vi "CSM - State Table - DebugTool.vi"() -> ()   [LabVIEW 2017]
doc: "<In Development> Real-time status table for the entire CSM program module."
uses:
  _Support/Typedef/_CSM_GlobalLog_MSG_TYPE.ctl
  _Support/Typedef/_CSM_GlobalLog_MSG.ctl
  _Support/Typedef/_CSM_Response Source Message.ctl
  _Polymophic/Add State(s) to Queue By BOOL(Element).vi
  76e8844a-bf39-49de-bef4-434369a066cd.vi
  e359954a-2527-40a5-9e0b-778f8f2f97ef.vi
  _Support/GlobalEvent/Gevt-ThreadQueueName.vi
  <vilib>/Utility/config.llb/Close Config Data.vi
  <vilib>/Utility/config.llb/Write Key.vi
  <vilib>/Utility/config.llb/Write Key (Double).vi
  <vilib>/Utility/config.llb/Write Key (I32).vi
  <vilib>/Utility/config.llb/Write Key (Path).vi
  <vilib>/Utility/config.llb/Write Key (String).vi
  <vilib>/Utility/config.llb/Write Key (Boolean).vi
  <vilib>/Utility/Data Type/Get Type Information.vi
  <vilib>/Utility/config.llb/Open Config Data.vi
  _csmHelper/lvcsmFile/lvcsm File Path.vi
  <vilib>/Utility/config.llb/Read Key.vi
  <vilib>/Utility/config.llb/Read Key (Double).vi
  <vilib>/Utility/config.llb/Read Key (I32).vi
  <vilib>/Utility/config.llb/Read Key (Path).vi
  <vilib>/Utility/config.llb/Read Key (String).vi
  <vilib>/Utility/config.llb/Read Key (Boolean).vi
  Communicable State Machine.lvlib
  _Support/csm-tool-support.lvlib
panel:
  in  "LogSize Limit:":i32=4 min=4 step=1
  out "ModuleNum:":i32=4 min=4 max=20 step=1
  out "LogSize:":i32=2 min=2 max=10 step=1
  in  "Content":string[][](array[string])
  in  "Row Header Strings[]":string[](array[string])
  in  "Exit":bool
  in  "Clear CSM":bool
  out "Table":string[][](table)
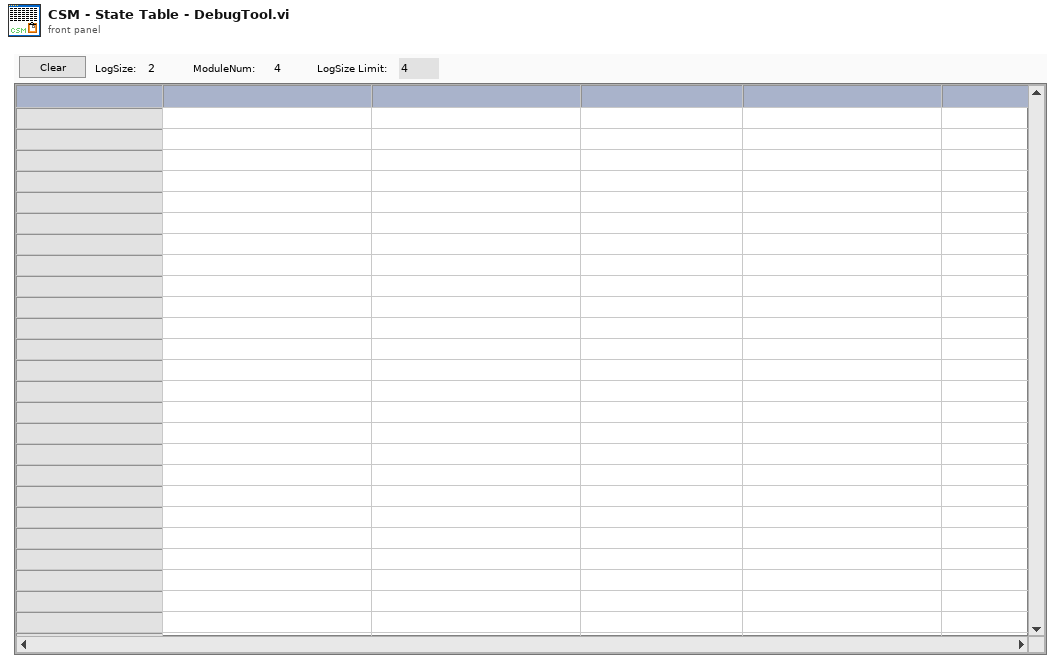
[diagram p1: front panel]
types:
  T1 = typedef "Communicable State Machine.lvlib/_CSM_GlobalLog_MSG_TYPE.ctl" = enum16{"User Log", "State Change", "Status", "Interrupt", "Register", "Unregister", "Error Log", "Module Created", "Module Destroyed"}
  T2 = enum32{"Invalid", "Standard", "Closed", "Hidden", "Minimized", "Maximized"}
  T3 = enum32{"invalid app kind", "Development System", "Run Time System", "Student Edition", "Embedded LabVIEW", "Evaluation", "Custom"}
  T4 = typedef "Communicable State Machine.lvlib/_CSM_GlobalLog_MSG.ctl" = cluster{"Name(\"\" to use uuid)":string, "Current State":string, "Arguments":string, "Source Message":T5, "Source Module":string, "Complete(T)/Start(F)":bool, "LogType":T1}
  T5 = typedef "Communicable State Machine.lvlib/_CSM_Response Source Message.ctl" = cluster{"‘State":string, "’Arguments":string, "’Error":errorcluster}
  T6 = cluster{"Core":cluster{"Current VI Reference":refnum<vi>, "Close Panel on Exit?":bool}, "Global-DataTable":string[][], "LogSize Limit":i32, "CSM Global Log Event":refnum<user-event>, "Log":T4, "LogTime":timestamp, "JKISM Names":string[], "RowHeaders":string[], "Content":string[][]}
  T7 = cluster{"Current VI Reference":refnum<vi>, "Close Panel on Exit?":bool}
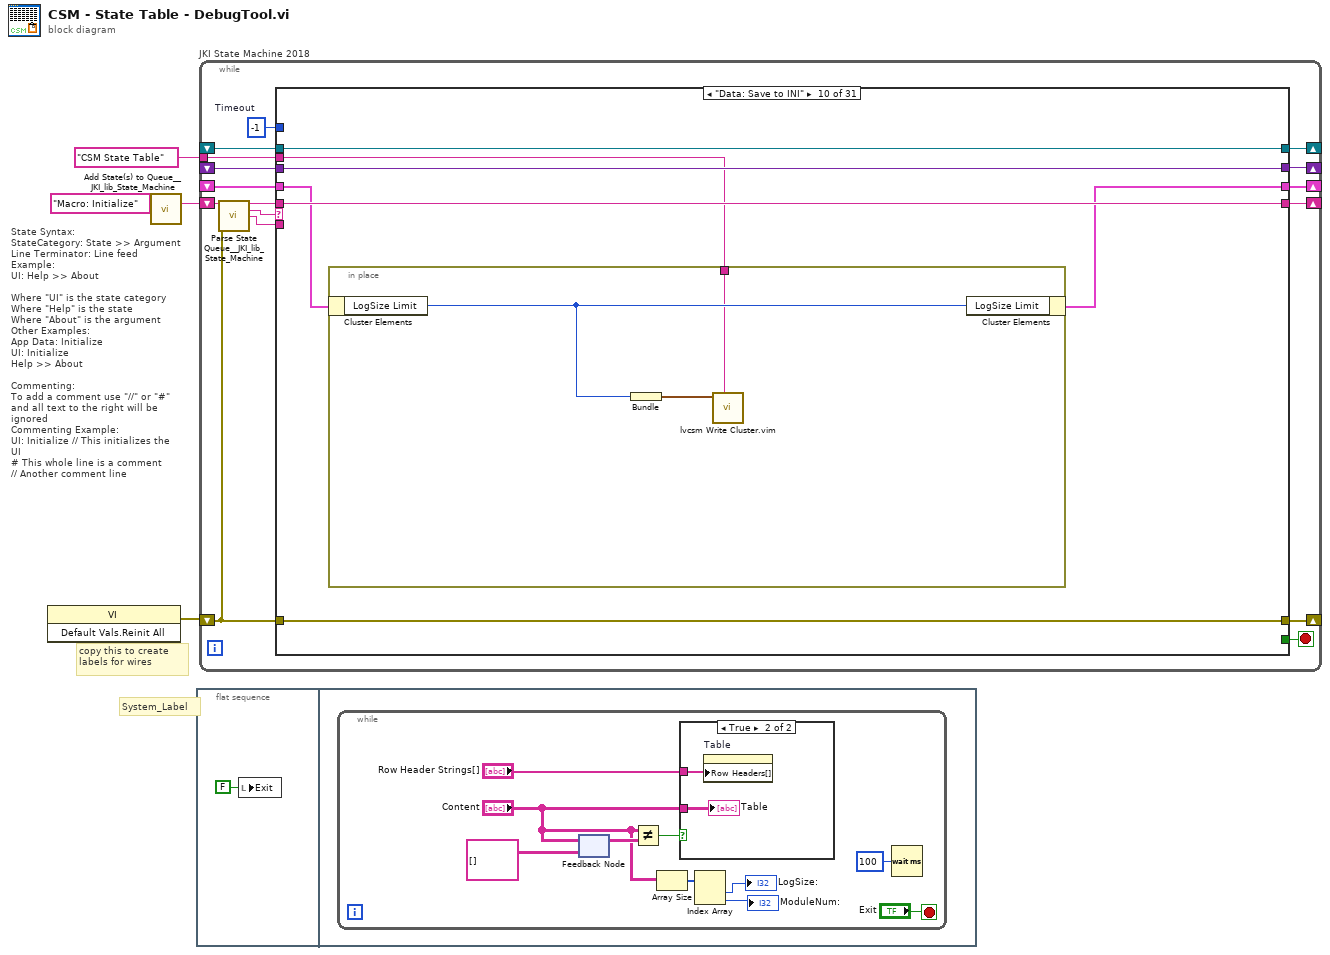
[diagram p0: block diagram]
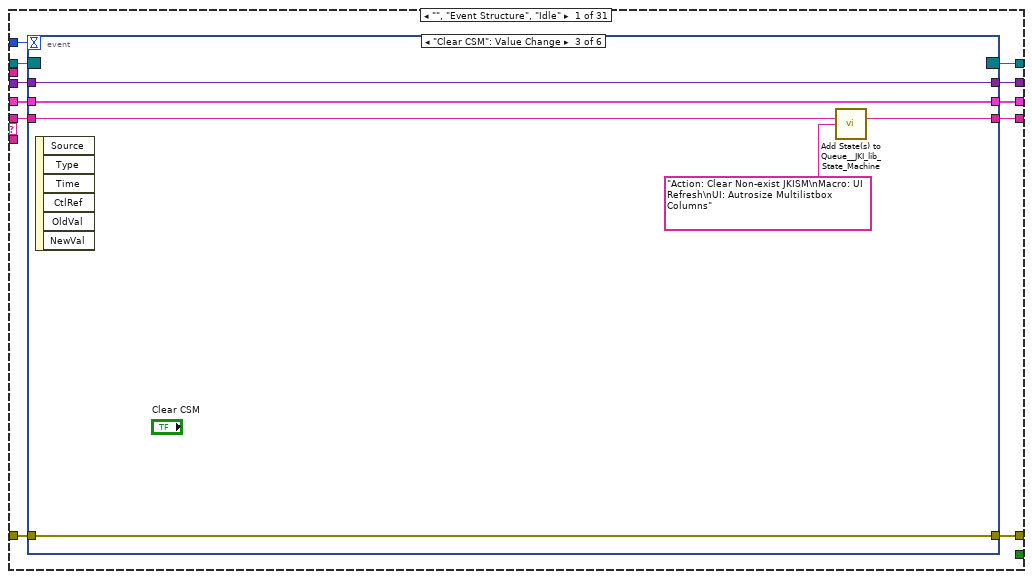
[diagram p3: hidden frame]
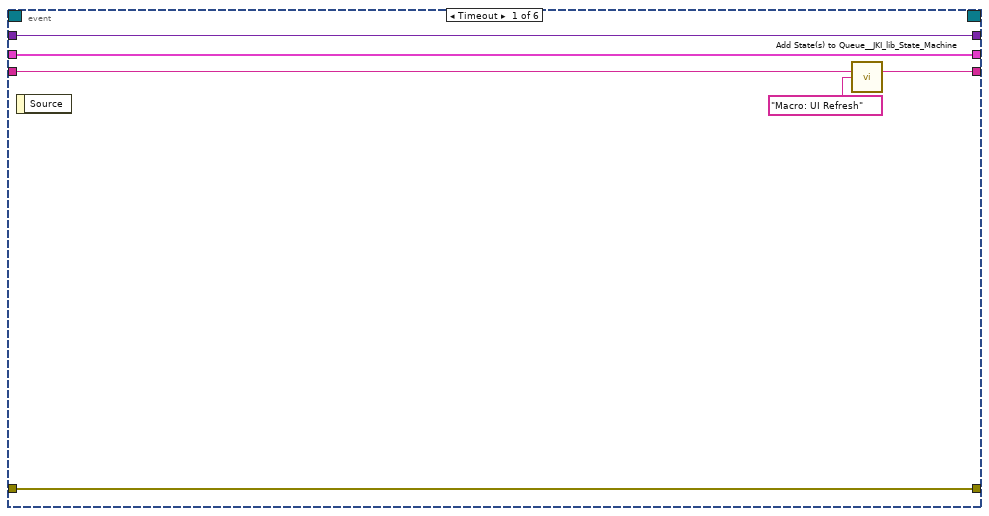
[diagram p4: hidden frame]
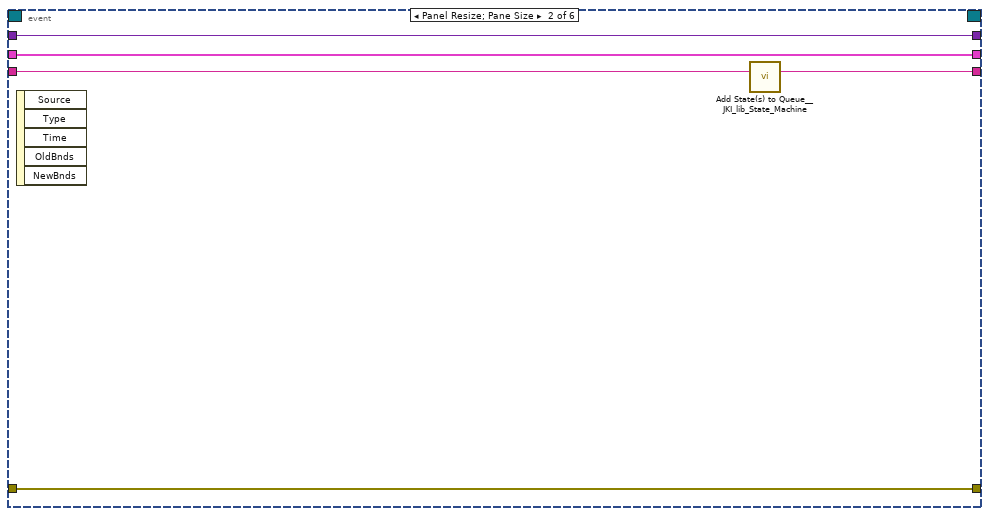
[diagram p5: hidden frame]
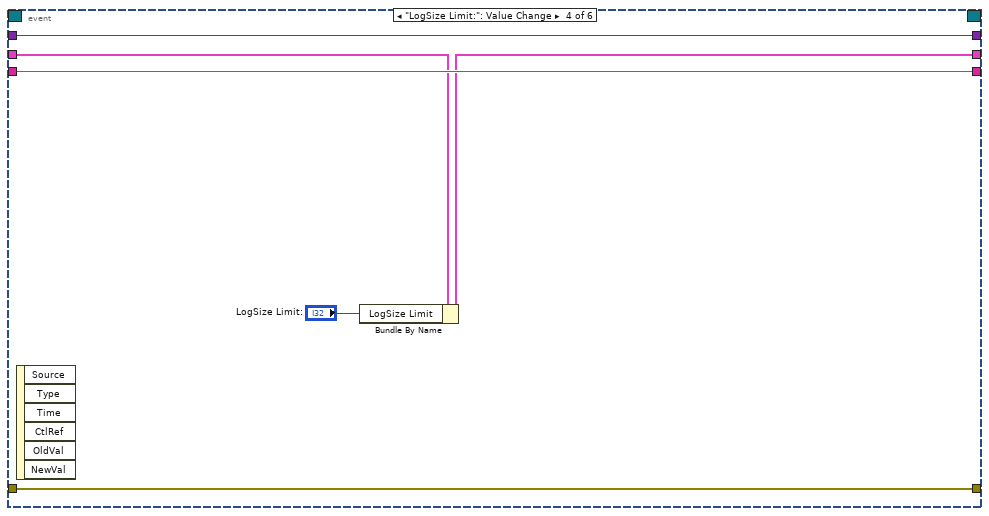
[diagram p6: hidden frame]
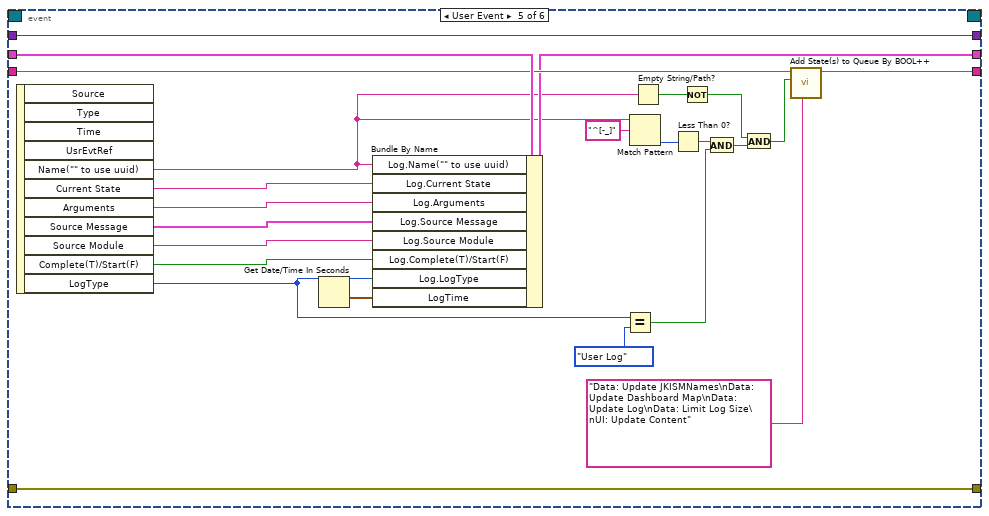
[diagram p7: hidden frame]
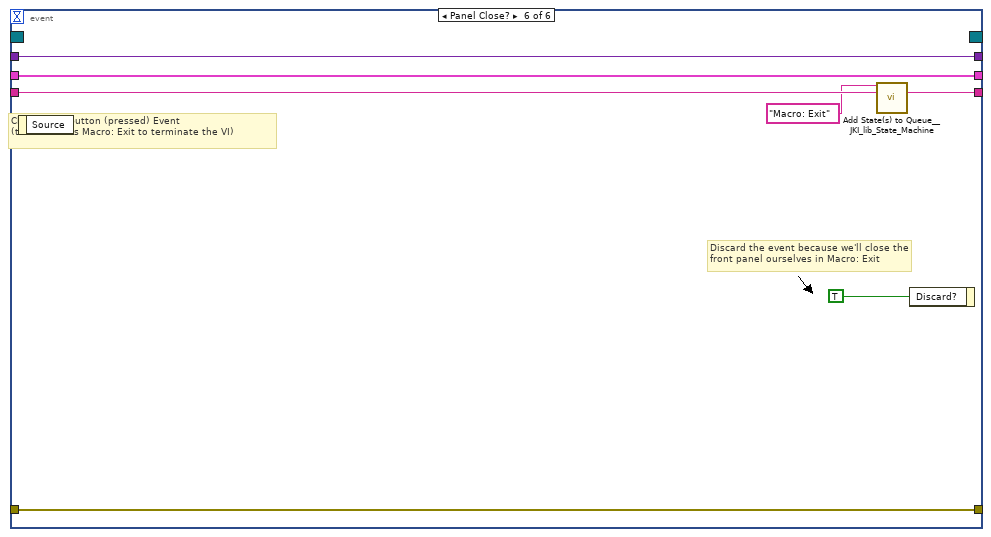
[diagram p8: hidden frame]
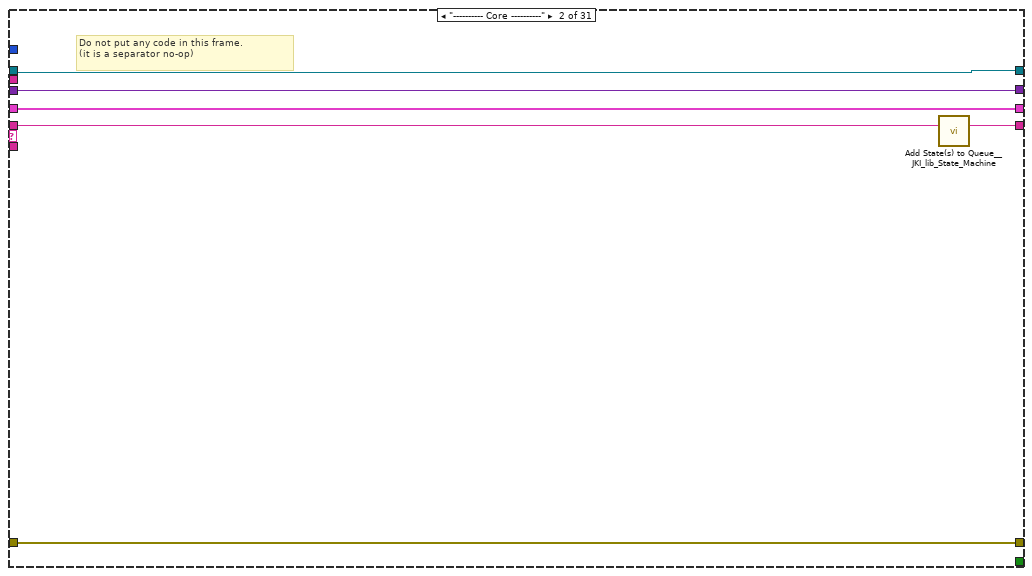
[diagram p9: hidden frame]
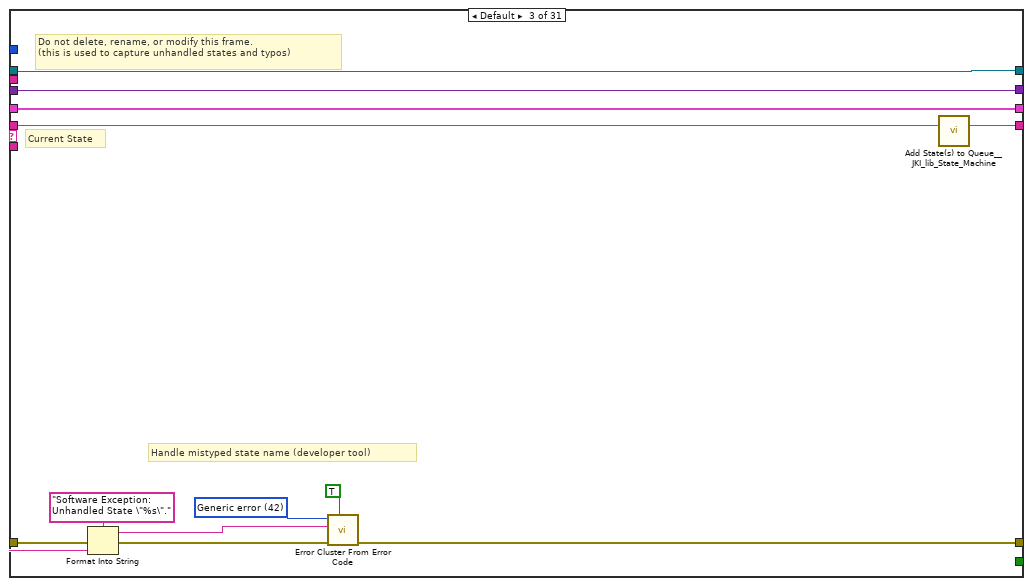
[diagram p10: hidden frame]
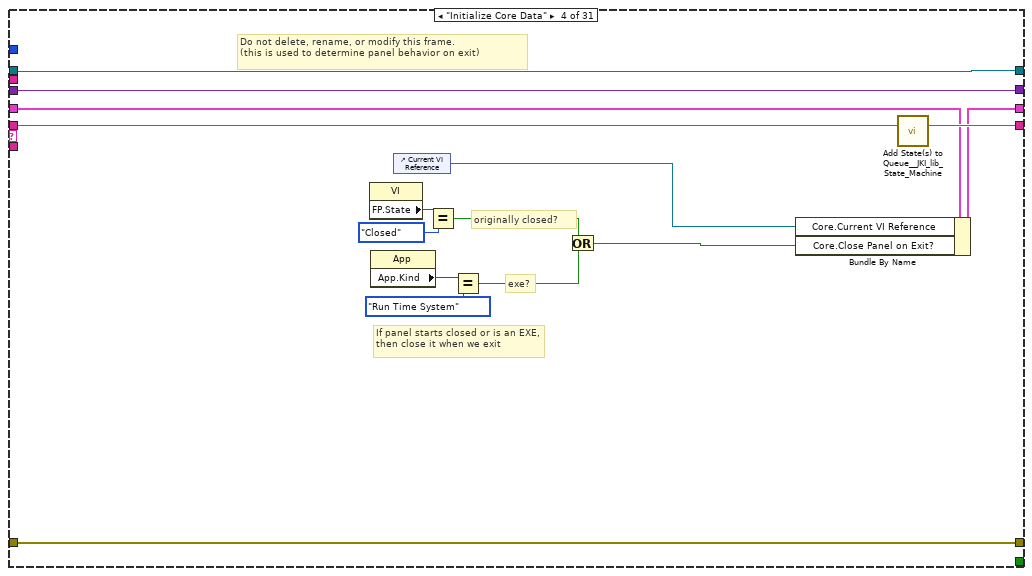
[diagram p11: hidden frame]
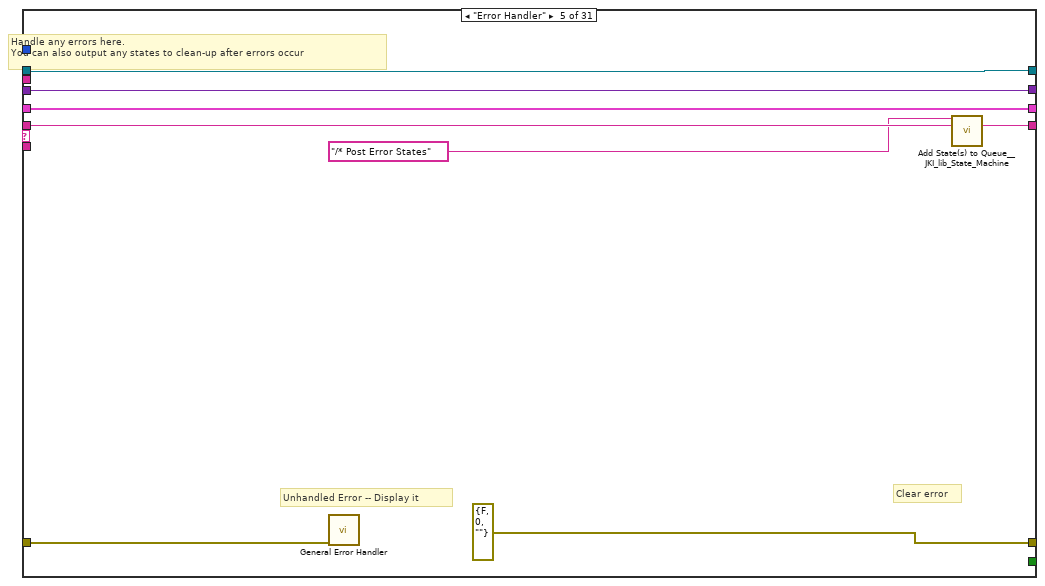
[diagram p12: hidden frame]
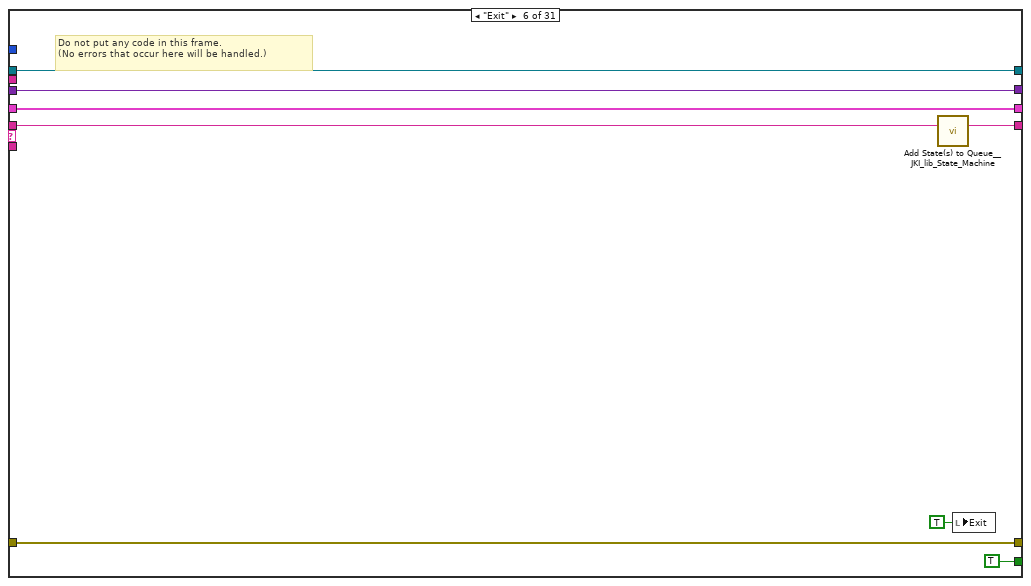
[diagram p13: hidden frame]
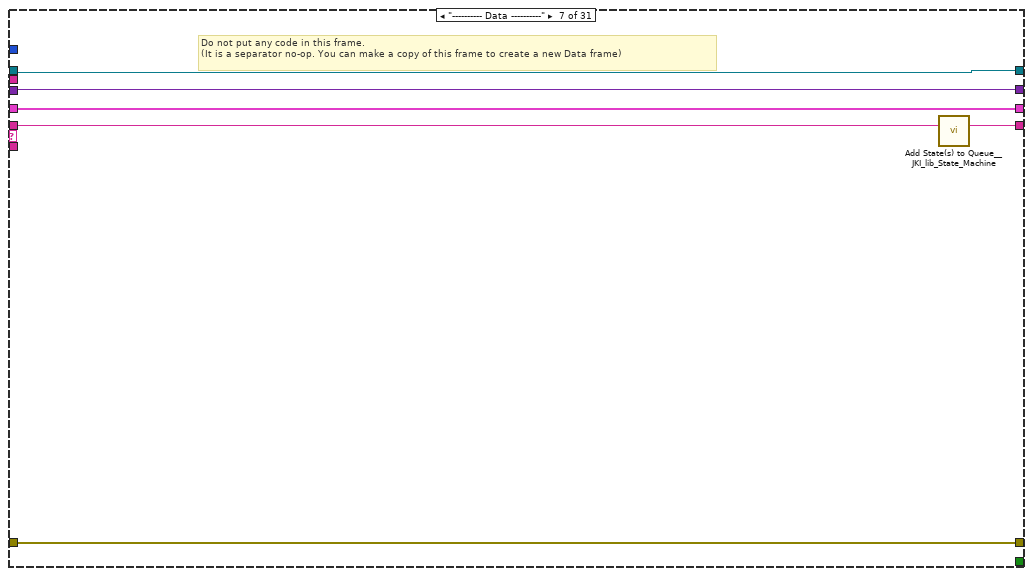
[diagram p14: hidden frame]
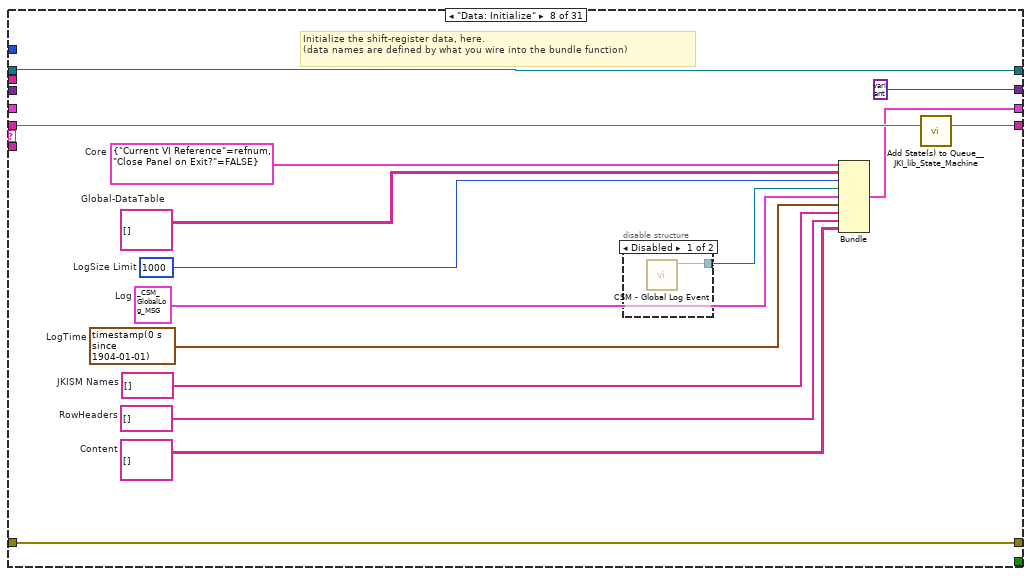
[diagram p15: hidden frame]
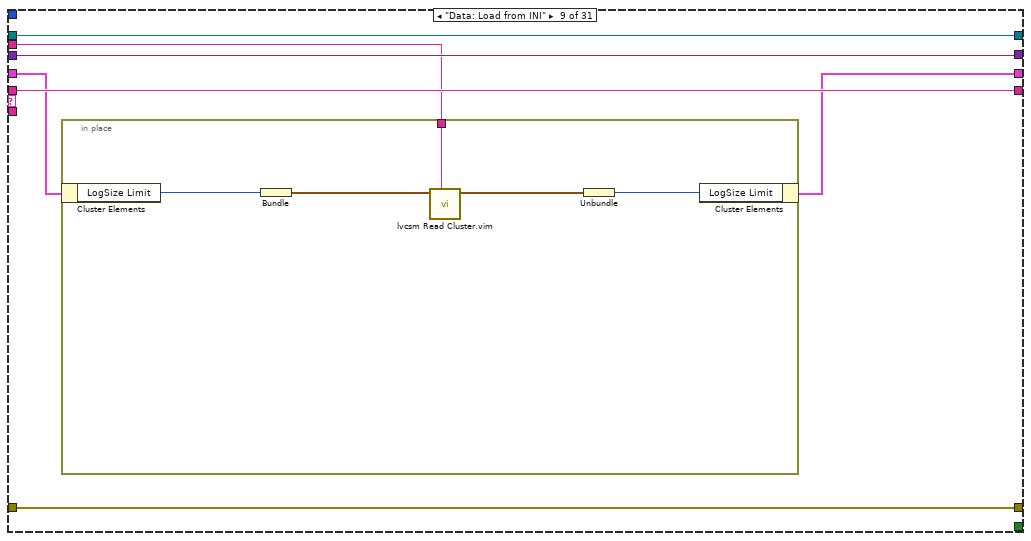
[diagram p17: hidden frame]
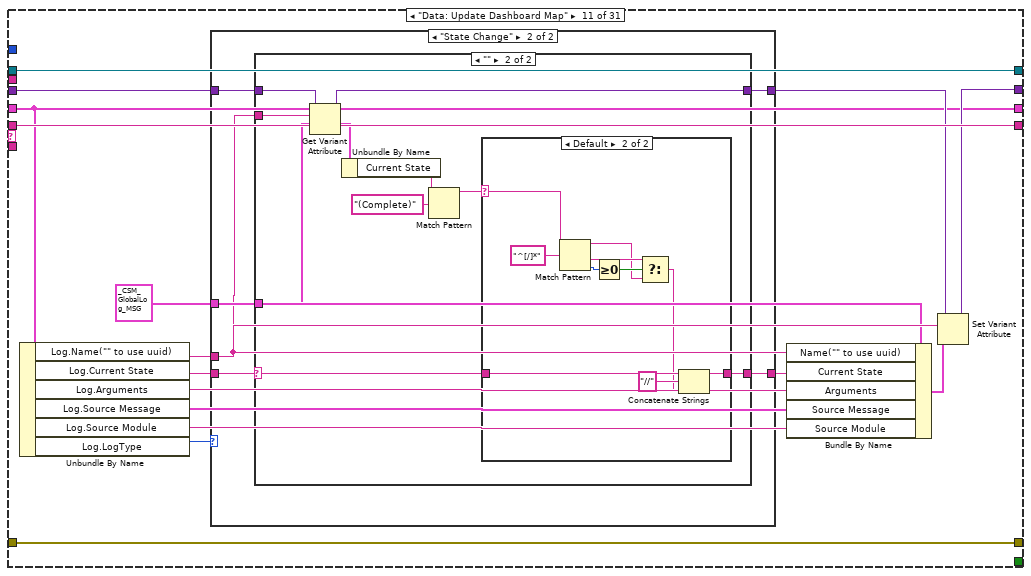
[diagram p18: hidden frame]
diagram:
  # "State Syntax:\nStateCategory: State >> Argument\nLine Terminator: Line feed\nExample:\nUI: Help >> About\n\nWhere \"UI\" is the state category\nWhere \"Help\" is the state\nWhere \"About\" is the argument\nOther Examples:\nApp Data: Initialize\nUI: Initialize\nHelp >> About\n\nCommenting:\nTo add a comment use \"//\" or \"#\" and all text to the right will be ignored\nCommenting Example:\nUI: Initialize // This initializes the UI\n# This whole line is a comment\n// Another comment line"
  # "copy this to create labels for wires"
  # "System_Label"
  n1 = invoke class="VI" method="Default Vals.Reinit All"() -> (error out=w2:errorcluster)  [unwired: 3 in, 2 out]
  n2 = call <vilib>:"Add State(s) to Queue__JKI_lib_State_Machine.vi"("State(s) in (\"\")"="Macro: Initialize") -> ("States Out"=w3:string)  [unwired: 14 in]
  n3 = flat-sequence {
    frame #0 {
      n4 = local write "Exit"(FALSE ("Exit")) -> ()
    }
    frame #1 {
      n5 = while {
        stop <- "Exit" stop-if-true
        n6 = feedback-in #1("Content") -> ()
        n7 = feedback #1(string[][] [] ("Content")) -> (w11:string[][])
        n8 = Not Equal?(x="Content", y=w11) -> (x != y?=w12:bool)
        n9 = Array Size(array="Content") -> (size(s)=w8:i32[])
        n10 = case shown="True" w12 {
          tunnel: "Content" -> [_ w17]
          tunnel: "Row Header Strings[]" -> [_ w16]
          frame False {
          }
          frame True {
            n11 = property on="Table" class="Tbl (strict)"("Row Headers[]"=w16) -> ()  [unwired: 2 in, 2 out]
            "Table" <- w17
          }
        }
        n12 = Index Array(array=w8) -> (element #1=→"LogSize:":i32, element #2=→"ModuleNum:":i32)  [unwired: 2 in]
        n13 = Wait (ms)(milliseconds to wait=u32 100) -> ()  [unwired: 1 out]
      }
    }
  }
  n14 = while "JKI State Machine 2018" {
    shift-right: [w26] -> _
    shift-left: _ -> [w25]
    shift-right: [w29] -> _
    shift-left: w2 -> [w23]
    shift-right: [w28] -> _
    shift-left: w3 -> [w30]
    shift-right: [w22] -> _
    shift-left: _ -> [w21]
    shift-right: [w20] -> _
    shift-left: _ -> [w19]
    tunnel: "CSM State Table" ("key") -> [w18]
    stop <- w27 stop-if-true
    w24 = -1  # Timeout
    n15 = call <vilib>:"Parse State Queue__JKI_lib_State_Machine.vi"("State Queue"=w30, "Error In (no error)"=w23) -> ("Remaining States"=w32:string, "Current State"=w33:string, "Arguments"=w31:string)  [unwired: 11 in]
    n16 = case shown="\"Data: Save to INI\"" w33 {
      selector: w33 -> [_ _ w107 _ _ _ _ _ _ _ _ _ _ _ _ _ _ _ _ _ _ _ _ _ _ _ _ _ _ _ _]
      tunnel: w32 -> [w44 w104 w111 w132 w140 w148 w154 w169 w176 w188 w207 w250 w281 w300 w316 w322 w330 w338 w351 w421 w428 w436 w440 w448 w456 w463 w470 w478 w491 w495 w520]
      tunnel: w31 -> [_ _ _ _ _ _ _ _ _ _ _ _ _ _ _ _ _ w333 w345 _ _ _ _ _ _ _ _ _ _ _ _]
      tunnel: w25 -> [w42 w101 w109 w125 w137 w146 w151 _ w175 w187 w195 w244 w277 w297 w311 w319 w324 w336 w347 w418 w425 w433 w439 w447 w452 w460 w467 w473 w488 w494 w511]
      tunnel: [w41 w102 w113 w129 errorcluster {"status"=FALSE, "code"=0, "source"=""} ("error out") w145 w152 w165 w177 w189 w208 w251 w282 w301 w310 w320 w328 w334 w348 w422 w429 w430 w441 w449 w457 w461 w468 w476 w489 w496 w521] -> w29
      tunnel: w23 -> [w40 w102 w112 w129 w136 w145 w152 w165 w177 w189 w208 w251 w282 w301 w313 w320 w328 w335 w349 w422 w429 _ w441 w449 w457 w461 w468 w476 w489 w496 w521]
      tunnel: [w43 w103 w110 w131 w139 w147 w153 w168 w176 w188 w207 w242 w281 w300 w315 w321 w329 w337 w350 w421 w428 w436 w440 w448 w456 w462 w469 w477 w490 w495 w520] -> w28
      tunnel: [_ _ _ _ _ TRUE _ _ _ _ _ _ _ _ _ _ _ _ _ _ _ _ _ _ _ _ _ _ _ _ _] -> w27
      tunnel: [w39 w101 w109 w130 w137 w146 w151 w167 w174 w186 w195 w243 w267 w296 w311 w319 w324 w336 w347 w418 w425 w433 w439 w443 w452 w460 w467 w473 w488 w494 w505] -> w26
      tunnel: w24 -> [w38 _ _ _ _ _ _ _ _ _ _ _ _ _ _ _ _ _ _ _ _ _ _ _ _ _ _ _ _ _ _]
      tunnel: [w36 w100 w106 w119 w134 w143 w150 variant w173 w185 w196 w248 w278 w299 w309 w318 w327 w332 w344 w420 w427 w435 w438 w446 w455 w459 w465 w472 w481 w493 w516] -> w22
      tunnel: w21 -> [w37 w100 w106 w119 w134 w143 w150 _ w173 w185 w197 w246 w279 w299 w309 w318 w327 w332 w344 w420 w427 w435 w438 w446 w455 w459 w465 w472 w481 w493 w518]
      tunnel: [w34 w99 w105 w118 w133 w142 w149 w161 w172 w184 w206 w249 w280 w298 w308 w317 w326 w331 w343 w419 w426 w434 w437 w444 w454 w458 w464 w471 w480 w492 w519] -> w20
      tunnel: w19 -> [w35 w99 w105 w118 w133 w142 w149 w161 w172 w184 w206 w249 w280 w298 w308 w317 w326 w331 w343 w419 w426 w434 w437 _ w454 w458 w464 w471 w480 w492 w519]
      tunnel: w18 -> [_ _ _ _ _ _ _ _ w171 w183 _ _ _ _ _ _ _ _ _ _ _ _ _ _ _ _ _ _ _ _ _]
      frame "", "Event Structure", "Idle" {
        n17 = event shown="[2] \"Clear CSM\": Value Change" {
          selector: w35 -> [_ _ _ _ _ _]
          dyn-events: [_ _ _ _ _ _] -> w34
          timeout: w38 -> [_ _ _ _ _ _]
          tunnel: w44 -> [w50 w52 w58 w67 w86 w98]
          tunnel: [w49 w53 w57 w67 w90 w97] -> w43
          tunnel: w42 -> [w47 w54 w60 w65 w87 w96]
          tunnel: [w48 w55 w61 w66 w91 w93] -> w41
          tunnel: w40 -> [w48 w55 w61 w66 w91 w93]
          tunnel: [w47 w54 w60 w63 w85 w96] -> w39
          tunnel: w37 -> [w45 w51 w59 w64 w88 w92]
          tunnel: [w45 w51 w59 w64 w88 w92] -> w36
          event Timeout {
            n18 = event-data() -> ()  [unwired: 1 in, 1 out]
            n19 = call <vilib>:"Add State(s) to Queue__JKI_lib_State_Machine.vi"("State(s) in (\"\")"=w50, "State(s) at Back (\"\")"="Macro: UI Refresh" ("State(s) in Front (\"\")")) -> ("States Out"=w49:string)  [unwired: 13 in]
          }
          event Panel Resize; Pane Size {
            n20 = event-data() -> ()  [unwired: 1 in, 5 out]
            n21 = call <vilib>:"Add State(s) to Queue__JKI_lib_State_Machine.vi"("State(s) in (\"\")"=w52) -> ("States Out"=w53:string)  [unwired: 14 in]
          }
          event "Clear CSM": Value Change {
            n22 = event-data() -> ()  [unwired: 1 in, 6 out]
            n23 = call <vilib>:"Add State(s) to Queue__JKI_lib_State_Machine.vi"("State(s) in (\"\")"=w58, "State(s) at Back (\"\")"="Action: Clear Non-exist JKISM\nMacro: UI Refresh\nUI: Autrosize Multilistbox Columns" ("State(s) at Back (\"\")")) -> ("States Out"=w57:string)  [unwired: 13 in]
          }
          event "LogSize Limit:": Value Change {
            n24 = event-data() -> ()  [unwired: 1 in, 6 out]
            n25 = Bundle By Name(cluster=w65, "LogSize Limit"="LogSize Limit:") -> (w63:T6)
          }
          event User Event {
            n26 = event-data() -> ("Name(\"\" to use uuid)"=w71:string, "Current State"=w80:string, "Arguments"=w81:string, "Source Message"=w82:T5, "Source Module"=w83:string, "Complete(T)/Start(F)"=w84:bool, "LogType"=w76:T1)  [unwired: 1 in, 4 out]
            n27 = Get Date/Time In Seconds() -> (seconds since 1Jan1904=w77:timestamp)
            n28 = Bundle By Name(cluster=w87, "Log.Name(\"\" to use uuid)"=w71, "Log.Current State"=w80, "Log.Arguments"=w81, "Log.Source Message"=w82, "Log.Source Module"=w83, "Log.Complete(T)/Start(F)"=w84, "Log.LogType"=w76, "LogTime"=w77) -> (w85:T6)
            n29 = Equal?(x=w76, y=_CSM_GlobalLog_MSG_TYPE."User Log") -> (x = y?=w73:bool)
            n30 = Match Pattern(string=w71, regular expression="^[-_]") -> (offset past match=w78:i32)  [unwired: 1 in, 3 out]
            n31 = Empty String/Path?(string/path=w71) -> (empty?=w69:bool)
            n32 = Less Than 0?(x=w78) -> (x < 0?=w74:bool)
            n33 = Not(x=w69) -> (.not. x?=w68:bool)
            n34 = And(x=w74, y=w73) -> (x .and. y?=w70:bool)
            n35 = And(x=w68, y=w70) -> (x .and. y?=w72:bool)
            n36 = call-poly "Add State(s) to Queue By BOOL++.vi"("TRUE(\"\")"="Data: Update JKISMNames\nData: Update Dashboard Map\nData: Update Log\nData: Limit Log Size\nUI: Update Content" ("State(s) at Back (\"\")"), "Condition"=w72, "State Queue(\"\")"=w86) -> ("Remaining States"=w90:string)  [unwired: 8 in]
          }
          event Panel Close? {
            # "Discard the event because we'll close the front panel ourselves in Macro: Exit"
            # "Close Panel button (pressed) Event\n(this executes Macro: Exit to terminate the VI)"
            n37 = event-data() -> ()  [unwired: 1 in, 1 out]
            n38 = call <vilib>:"Add State(s) to Queue__JKI_lib_State_Machine.vi"("State(s) in Front (\"\")"="Macro: Exit", "State(s) in (\"\")"=w98) -> ("States Out"=w97:string)  [unwired: 13 in]
            n39 = event-data("Discard?"=TRUE) -> ()  [unwired: 1 in, 1 out]
          }
        }
      }
      frame "---------- Core ----------" {
        # "Do not put any code in this frame.\n(it is a separator no-op)"
        n40 = call <vilib>:"Add State(s) to Queue__JKI_lib_State_Machine.vi"("State(s) in (\"\")"=w104) -> ("States Out"=w103:string)  [unwired: 14 in]
      }
      frame Default {
        w116 = 42 items=["No error", "Argument error", "Memory is full", "Out of zone", "End of file", "File already open", "Generic file I/O error", "File not found", "File permission error", "Disk is full", "Duplicate path", "Too many files open", "System feature not enabled", "Resource file not found", "Cannot add resource", "Resource not found", "Image not found", "Image memory error", "Pen does not exist", "Config type invalid", "Config token not found", "Config parse error", "Config memory error", "Bad external code format", "Bad external code offset", "External code not present", "Null window", "Destroy window error", "Null menu", "Print aborted", "Bad print record", "Print driver error", "Windows error during printing", "Memory error during printing", "Print dialog error", "Generic print error", "Invalid device refnum", "Device not found", "Device parameter error", "Device unit error", "Cannot open device", "Device call aborted", "Generic error", "Cancelled by user", "Object ID too low", "Object ID too high", "Object not in heap", "Unknown heap", "Unknown object (invalid DefProc)", "Unknown object (DefProc not in table)", "Message out of range", "Invalid (null) method", "Unknown message", "Manager call not supported", "Bad address", "Network operation in progress", "Network operation timed out", "Connection is busy", "Network attribute not supported", "Network error", "Address in use", "System out of memory", "Connection aborted", "Connection refused", "Not connected", "Already connected", "Connection closed", "Initialization error (interapplication manager)", "Bad occurrence", "Wait on unbound occurrence handler", "Occurrence queue overflow", "Datalog type conflict", "Unused", "Unrecognized type (interapplication manager)", "Memory corrupt", "Failed to make temporary DLL", "Old CIN version", "Drag socket not found", "Failed to load drop-object", "Failed to register OLE object", "Failed to release OLE object", "Format specifier type mismatch", "Unknown format specifier", "Too few format specifiers", "Too many format specifiers", "Scan failed", "Newer CIN version", "Error converting to variant", "Runtime menu error", "Password tampered", "Variant attribute not found", "Incompatible variant data type", "Event data is not available", "Event Store is not present", "Occurrence is not found", "Event Queue is not created", "Event info is not available", "Refnum passed is NULL", "Error retrieving Class GUID", "Error retrieving CoClass GUID", "Error retrieving TypeLib GUID.", "Bad built application magic bytes.", "Specific driver is different from the specific driver associated with the Logical Name.", "There is no session opened to the class driver.", "Max Error", "MAX - Error with config objects", "MAX - Error loading configuration", "MAX - Group not supported"]
        # "Current State"
        # "Do not delete, rename, or modify this frame.\n(this is used to capture unhandled states and typos)"
        # "Handle mistyped state name (developer tool)"
        n41 = Format Into String(format string="Software Exception: Unhandled State \"%s\"." ("message"), error in=w112, w107) -> (resulting string=w115:string, error out=w114:errorcluster)  [unwired: 1 in]
        n42 = call <vilib>:"Error Cluster From Error Code.vi"("show call chain? (False)"=TRUE, "error in (no error)"=w114, "error message (\"\")"=w115, "error code (0)"=w116) -> ("error out"=w113:errorcluster)  [unwired: 5 in]
        n43 = call <vilib>:"Add State(s) to Queue__JKI_lib_State_Machine.vi"("State(s) in (\"\")"=w111) -> ("States Out"=w110:string)  [unwired: 14 in]
      }
      frame "Initialize Core Data" {
        # "Do not delete, rename, or modify this frame.\n(this is used to determine panel behavior on exit)"
        # "originally closed?"
        # "exe?"
        # "If panel starts closed or is an EXE, then close it when we exit"
        n44 = property class="VI"() -> ("FP.State"=w122:T2)  [unwired: 2 in, 2 out]
        n45 = property class="App"() -> ("App.Kind"=w128:T3)  [unwired: 2 in, 2 out]
        n46 = control-ref of="Current VI Reference"() -> (w123:refnum<vi>)
        n47 = Equal?(x=w122, y=T2."Closed" ("Front Panel Window:State")) -> (x = y?=w120:bool)
        n48 = Equal?(x=w128, y=T3."Run Time System" ("Application:Kind")) -> (x = y?=w126:bool)
        n49 = Or(x=w120, y=w126) -> (x .or. y?=w124:bool)
        n50 = Bundle By Name(cluster=w125, "Core.Current VI Reference"=w123, "Core.Close Panel on Exit?"=w124) -> (w130:T6)
        n51 = call <vilib>:"Add State(s) to Queue__JKI_lib_State_Machine.vi"("State(s) in (\"\")"=w132) -> ("States Out"=w131:string)  [unwired: 14 in]
      }
      frame "Error Handler" {
        # "Unhandled Error -- Display it"
        # "Handle any errors here.\nYou can also output any states to clean-up after errors occur"
        # "Clear error"
        n52 = call <vilib>:"General Error Handler.vi"("error in (no error)"=w136) -> ()  [unwired: 10 in, 5 out]
        n53 = call <vilib>:"Add State(s) to Queue__JKI_lib_State_Machine.vi"("State(s) in Front (\"\")"="/* Post Error States", "State(s) in (\"\")"=w140) -> ("States Out"=w139:string)  [unwired: 13 in]
      }
      frame "Exit" {
        # "Do not put any code in this frame.\n(No errors that occur here will be handled.)"
        n54 = call <vilib>:"Add State(s) to Queue__JKI_lib_State_Machine.vi"("State(s) in (\"\")"=w148) -> ("States Out"=w147:string)  [unwired: 14 in]
        n55 = local write "Exit"(TRUE ("Exit")) -> ()
      }
      frame "---------- Data ----------" {
        # "Do not put any code in this frame.\n(It is a separator no-op. You can make a copy of this frame to create a new Data frame)"
        n56 = call <vilib>:"Add State(s) to Queue__JKI_lib_State_Machine.vi"("State(s) in (\"\")"=w154) -> ("States Out"=w153:string)  [unwired: 14 in]
      }
      frame "Data: Initialize" {
        w155 = string[][] []  # Content
        w156 = string[] []  # RowHeaders
        w157 = timestamp(0 s since 1904-01-01)  # LogTime
        w158 = string[] []  # JKISM Names
        w159 = T4 {"Name(\"\" to use uuid)"="", "Current State"="", "Arguments"="", "Source Message"={"‘State"="", "’Arguments"="", "’Error"={"status"=FALSE, "code"=0, "source"=""}}, "Source Module"="", "Complete(T)/Start(F)"=FALSE, "LogType"=enum."User Log"}  # Log
        w163 = 1000  # LogSize Limit
        w164 = string[][] []  # Global-DataTable
        w166 = T7 {"Current VI Reference"=refnum, "Close Panel on Exit?"=FALSE}  # Core
        # "Initialize the shift-register data, here.\n(data names are defined by what you wire into the bundle function)"
        n57 = disable-structure shown="Disabled" {
          disable-tunnel: [w170 _] -> w160
          frame Disabled {
            n58 = call "CSM - Global Log Event.vi"() -> ("CSM Global Log Event"=w170:refnum<user-event>)  [unwired: 10 in, 1 out]
          }
          frame Enabled {
          }
        }
        n59 = Bundle("Core"=w166, "Global-DataTable"=w164, "LogSize Limit"=w163, "CSM Global Log Event"=w160, "Log"=w159, "LogTime"=w157, "JKISM Names"=w158, "RowHeaders"=w156, "Content"=w155) -> (w167:T6)  [unwired: 1 in]
        n60 = call <vilib>:"Add State(s) to Queue__JKI_lib_State_Machine.vi"("State(s) in (\"\")"=w169) -> ("States Out"=w168:string)  [unwired: 14 in]
      }
      frame "Data: Load from INI" {
        n61 = in-place {
          in-place-border: w171 -> [w180]
          n62 = in-place-cluster #2(w175) -> ("LogSize Limit"=w182:i32)
          n63 = Bundle("LogSize Limit"=w182) -> (w179:cluster{"LogSize Limit":i32})  [unwired: 1 in]
          n64 = call "lvcsm Read Cluster.vim"("Section"=w180, "Default Prototype"=w179) -> ("Cluster (dup)"=w181:cluster{"LogSize Limit":i32})  [unwired: 8 in, 1 out]
          n65 = Unbundle(w181) -> ("LogSize Limit"=w178:i32)
          n66 = in-place-cluster #2("LogSize Limit"=w178) -> (w174:T6)
        }
      }
      frame "Data: Save to INI" {
        n67 = in-place {
          in-place-border: w183 -> [w191]
          n68 = in-place-cluster #3(w187) -> ("LogSize Limit"=w192:i32)
          n69 = Bundle("LogSize Limit"=w192) -> (w190:cluster{"LogSize Limit":i32})  [unwired: 1 in]
          n70 = call "lvcsm Write Cluster.vim"("Section"=w191, "Default Prototype"=w190) -> ()  [unwired: 9 in, 1 out]
          n71 = in-place-cluster #3("LogSize Limit"=w192) -> (w186:T6)
        }
      }
      frame "Data: Update Dashboard Map" {
        w198 = T4 {"Name(\"\" to use uuid)"="", "Current State"="", "Arguments"="", "Source Message"={"‘State"="", "’Arguments"="", "’Error"={"status"=FALSE, "code"=0, "source"=""}}, "Source Module"="", "Complete(T)/Start(F)"=FALSE, "LogType"=enum."User Log"} ("Cross JKI State Machine Data")
        n72 = Unbundle By Name(w195) -> ("Log.Name(\"\" to use uuid)"=w199:string, "Log.Current State"=w194:string, "Log.Arguments"=w201:string, "Log.Source Message"=w202:T5, "Log.Source Module"=w203:string, "Log.LogType"=w193:T1)
        n73 = case shown="\"State Change\"" w193 {
          tunnel: [w210 w216] -> w204
          tunnel: [w209 w215] -> w200
          tunnel: w199 -> [_ w214]
          tunnel: w198 -> [_ w213]
          tunnel: w197 -> [w210 w212]
          tunnel: w194 -> [w209 w211]
          frame "User Log", Default {
          }
          frame "State Change" {
            n74 = case shown="\"\"" w211 {
              selector: w211 -> [w217 w220]
              tunnel: w212 -> [w218 w228]
              tunnel: [w218 w227] -> w216
              tunnel: w214 -> [_ w226]
              tunnel: w213 -> [_ w224]
              tunnel: [w217 w219] -> w215
              frame Default {
              }
              frame "" {
                n75 = Get Variant Attribute(Variant=w228, name=w226, default value (empty Variant)=w224) -> (duplicate Variant=w227:variant, value=w225:T4)  [unwired: 1 in, 2 out]
                n76 = Unbundle By Name(w225) -> ("Current State"=w223:string)
                n77 = Match Pattern(string=w223, regular expression="(Complete)") -> (before substring=w221:string)  [unwired: 1 in, 3 out]
                n78 = case shown="Default" w221 {
                  selector: w221 -> [_ w235]
                  tunnel: w220 -> [w229 w239]
                  tunnel: [w229 w238] -> w219
                  frame "" {
                  }
                  frame Default {
                    n79 = Match Pattern(string=w235, regular expression="^[/]*") -> (before substring=w230:string, after substring=w232:string, offset past match=w234:i32)  [unwired: 1 in, 1 out]
                    n80 = Greater Or Equal To 0?(x=w234) -> (x >= 0?=w233:bool)
                    n81 = Select(t=w232, s=w233, f=w230) -> (s? t:f=w231:string)
                    n82 = Concatenate Strings(w239, "//" ("string"), w231) -> (w238:string)
                  }
                }
              }
            }
          }
        }
        n83 = Bundle By Name(cluster=w198, "Name(\"\" to use uuid)"=w199, "Current State"=w200, "Arguments"=w201, "Source Message"=w202, "Source Module"=w203) -> (w205:T4)
        n84 = Set Variant Attribute(Variant=w204, name=w199, value=w205) -> (Variant out=w196:variant)  [unwired: 1 in, 2 out]
      }
      frame "Data: Update JKISMNames" {
        n85 = Unbundle By Name(w244) -> ("Log.Name(\"\" to use uuid)"=w245:string)
        n86 = Get Variant Attribute(Variant=w246, name=w245, default value (empty Variant)=T4 {"Name(\"\" to use uuid)"="", "Current State"="", "Arguments"="", "Source Message"={"‘State"="", "’Arguments"="", "’Error"={"status"=FALSE, "code"=0, "source"=""}}, "Source Module"="", "Complete(T)/Start(F)"=FALSE, "LogType"=enum."User Log"} ("Cross JKI State Machine Data")) -> (duplicate Variant=w248:variant, found=w241:bool)  [unwired: 1 in, 2 out]
        n87 = case shown="False" w241 {
          tunnel: w244 -> [w254 w257]
          tunnel: w245 -> [w255 _]
          tunnel: [w252 w257] -> w243
          frame False {
            n88 = Unbundle By Name(w254) -> ("JKISM Names"=w256:string[])
            n89 = Build Array (concatenate)(w256, w255) -> (w253:string[])
            n90 = Bundle By Name(cluster=w254, "JKISM Names"=w253) -> (w252:T6)
          }
          frame True {
          }
        }
        n91 = call-poly "Add State(s) to Queue By BOOL++.vi"("FALSE(\"\")"="UI: Update Column Names" ("TRUE(\"\")"), "Condition"=w241, "State Queue(\"\")"=w250) -> ("Remaining States"=w242:string)  [unwired: 8 in]
      }
      frame "Data: Update Log" {
        n92 = Unbundle By Name(w277) -> ("Content"=w268:string[][], "JKISM Names"=w276:string[], "RowHeaders"=w265:string[], "LogTime"=w259:timestamp)
        n93 = for {
          shift-right: [w293] -> w278
          shift-left: w279 -> [w294]
          tunnel: w276 -> [w292] mode=indexing
          tunnel: [w290] -> w274 mode=indexing
          n94 = Get Variant Attribute(Variant=w294, name=w292, default value (empty Variant)=T4 {"Name(\"\" to use uuid)"="", "Current State"="", "Arguments"="", "Source Message"={"‘State"="", "’Arguments"="", "’Error"={"status"=FALSE, "code"=0, "source"=""}}, "Source Module"="", "Complete(T)/Start(F)"=FALSE, "LogType"=enum."User Log"} ("Cross JKI State Machine Data")) -> (duplicate Variant=w293:variant, value=w291:T4)  [unwired: 1 in, 2 out]
          n95 = Unbundle By Name(w291) -> ("Current State"=w290:string)
        }
        n96 = Get Date/Time String(seconds (now)=w259, want seconds? (F)=TRUE) -> (date string=w262:string, time string=w261:string)  [unwired: 1 in]
        n97 = Concatenate Strings(w262, " " ("string"), w261) -> (w258:string)
        n98 = Array Size(array=w268) -> (size(s)=w275:i32[])
        n99 = Array Size(array=w274) -> (size(s)=w273:i32)
        n100 = Index Array(array=w275) -> (element #1=w272:i32, element #2=w271:i32)  [unwired: 2 in]
        n101 = Greater?(x=w273, y=w271) -> (0:w269:bool)
        n102 = case shown="True" w269 {
          tunnel: w268 -> [w283 w289]
          tunnel: w272 -> [_ w287]
          tunnel: w271 -> [_ w285]
          tunnel: [w283 w284] -> w270
          frame False {
          }
          frame True {
            n103 = Initialize Array("" ("Current State"), w287) -> (w286:string[])
            n104 = Insert Into Array(array=w289, index (col)=w285, new element=w286) -> (w284:string[][])  [unwired: 1 in]
          }
        }
        n105 = Build Array (concatenate)(w258, w265) -> (w264:string[])
        n106 = Build Array (concatenate)(w274, w270) -> (w266:string[][])
        n107 = Bundle By Name(cluster=w277, "Content"=w266, "RowHeaders"=w264) -> (w267:T6)
      }
      frame "Data: Limit Log Size" {
        n108 = in-place {
          w303 = 0 ("index")
          n109 = in-place-cluster #4(w297) -> ("Content"=w305:string[][], "RowHeaders"=w306:string[], "LogSize Limit"=w302:i32)
          n110 = Array Subset(array=w305, index (row)=w303, length (row)=w302) -> (w304:string[][])  [unwired: 2 in]
          n111 = Array Subset(array=w306, index=w303, length=w302) -> (w307:string[])
          n112 = in-place-cluster #4("Content"=w304, "RowHeaders"=w307, "LogSize Limit"=w302) -> (w296:T6)
        }
      }
      frame "Data: Cleanup" {
        # "Cleanup any data and references, here.\n(this is called automatically, by the Macro: Exit)"
        n113 = Unbundle By Name(w311) -> ("Core.Current VI Reference"=w314:refnum<vi>)
        n114 = Close Reference(reference=w314, error in (no error)=w313) -> (error out=w312:errorcluster)
        n115 = Merge Errors(w312) -> (w310:errorcluster)
        n116 = call <vilib>:"Add State(s) to Queue__JKI_lib_State_Machine.vi"("State(s) in (\"\")"=w316) -> ("States Out"=w315:string)  [unwired: 14 in]
      }
      frame "---------- UI ----------" {
        # "Do not put any code in this frame.\n(It is a separator no-op. You can make a copy of this frame to create a new UI frame)"
        n117 = call <vilib>:"Add State(s) to Queue__JKI_lib_State_Machine.vi"("State(s) in (\"\")"=w322) -> ("States Out"=w321:string)  [unwired: 14 in]
      }
      frame "UI: Initialize" {
        # "Initialize the User Interface, here.\n(this is called automatically, by the Macro: Init)"
        n118 = Unbundle By Name(w324) -> ("LogSize Limit"=w323:i32)
        n119 = property on="Table" class="Tbl (strict)"("Row Headers[]"=string[] [] ("Row Header Strings[]")) -> ()  [unwired: 2 in, 2 out]
        n120 = local write "LogSize Limit:"(w323) -> ()
        n121 = call <vilib>:"Add State(s) to Queue__JKI_lib_State_Machine.vi"("State(s) in (\"\")"=w330) -> ("States Out"=w329:string)  [unwired: 14 in]
      }
      frame "UI: Cursor Set" {
        # "Argument"
        # "Set and Unset Cursor Busy.\n(Usage: \"UI: Cursor Set >> Busy|Idle\")"
        n122 = case shown="\"Idle\", Default" w333 {
          tunnel: w335 -> [w340 w342]
          tunnel: [w339 w341] -> w334
          frame "Idle", Default {
            n123 = call <vilib>:"Unset Busy.vi"("error in (no error)"=w340) -> ("error out"=w339:errorcluster)  [unwired: 10 in]
          }
          frame "Busy" {
            n124 = call <vilib>:"Set Busy.vi"("error in (no error)"=w342) -> ("error out"=w341:errorcluster)  [unwired: 9 in, 1 out]
          }
        }
        n125 = call <vilib>:"Add State(s) to Queue__JKI_lib_State_Machine.vi"("State(s) in (\"\")"=w338) -> ("States Out"=w337:string)  [unwired: 14 in]
      }
      frame "UI: Front Panel State" {
        # "Argument"
        # "Set Front Panel Open or Closed\n(Usage: \"UI: Front Panel State >> Open|Close\")"
        n126 = Unbundle By Name(w347) -> ("Core.Current VI Reference"=w346:refnum<vi>)
        n127 = case shown="\"Minimize\", \"Minimized\"" w345 {
          tunnel: w349 -> [w357 w372 w383 w396 w409]
          tunnel: [w359 w373 w385 w398 w411] -> w348
          tunnel: w346 -> [w358 w370 w384 w397 w410]
          frame "Open", "Standard", Default {
            w352 = T2."Standard" ("State")
            n128 = property class="VI"(reference=w358, error in=w357) -> (reference out=w355:refnum<vi>, error out=w356:errorcluster, "FP.State"=w354:T2)
            n129 = Not Equal?(x=w354, y=w352) -> (x != y?=w353:bool)
            n130 = case shown="True" w353 {
              tunnel: [w363 w365] -> w359
              tunnel: w356 -> [w362 w365]
              tunnel: w355 -> [w361 _]
              tunnel: w352 -> [w360 _]
              frame True {
                n131 = invoke class="VI" method="FP.Open"(reference=w361, error in=w362, "Activate"=TRUE, "State"=w360) -> (error out=w363:errorcluster)  [unwired: 1 in, 4 out]
              }
              frame False {
              }
            }
          }
          frame "Close", "Closed" {
            n132 = property class="VI"(reference=w370, error in=w372) -> (reference out=w369:refnum<vi>, error out=w371:errorcluster, "FP.State"=w367:T2)
            n133 = Not Equal?(x=w367, y=T2."Closed" ("Front Panel Window:State")) -> (x != y?=w366:bool)
            n134 = case shown="True" w366 {
              tunnel: [w374 w377] -> w373
              tunnel: w371 -> [w374 w376]
              tunnel: w369 -> [_ w375]
              frame False {
              }
              frame True {
                n135 = invoke class="VI" method="FP.Close"(reference=w375, error in=w376) -> (error out=w377:errorcluster)  [unwired: 1 in, 2 out]
              }
            }
          }
          frame "Hidden", "Hide" {
            w378 = T2."Hidden" ("State")
            n136 = property class="VI"(reference=w384, error in=w383) -> (reference out=w381:refnum<vi>, error out=w382:errorcluster, "FP.State"=w380:T2)
            n137 = Not Equal?(x=w380, y=w378) -> (x != y?=w379:bool)
            n138 = case shown="True" w379 {
              tunnel: [w389 w390] -> w385
              tunnel: w382 -> [w388 w390]
              tunnel: w381 -> [w387 _]
              tunnel: w378 -> [w386 _]
              frame True {
                n139 = invoke class="VI" method="FP.Open"(reference=w387, error in=w388, "State"=w386) -> (error out=w389:errorcluster)  [unwired: 2 in, 4 out]
              }
              frame False {
              }
            }
          }
          frame "Minimize", "Minimized" {
            w391 = T2."Minimized" ("State")
            n140 = property class="VI"(reference=w397, error in=w396) -> (reference out=w394:refnum<vi>, error out=w395:errorcluster, "FP.State"=w393:T2)
            n141 = Not Equal?(x=w393, y=w391) -> (x != y?=w392:bool)
            n142 = case shown="True" w392 {
              tunnel: [w402 w403] -> w398
              tunnel: w395 -> [w401 w403]
              tunnel: w394 -> [w400 _]
              tunnel: w391 -> [w399 _]
              frame True {
                n143 = invoke class="VI" method="FP.Open"(reference=w400, error in=w401, "State"=w399) -> (error out=w402:errorcluster)  [unwired: 2 in, 4 out]
              }
              frame False {
              }
            }
          }
          frame "Maximize", "Maximized" {
            w404 = T2."Maximized" ("State")
            n144 = property class="VI"(reference=w410, error in=w409) -> (reference out=w407:refnum<vi>, error out=w408:errorcluster, "FP.State"=w406:T2)
            n145 = Not Equal?(x=w406, y=w404) -> (x != y?=w405:bool)
            n146 = case shown="True" w405 {
              tunnel: [w415 w416] -> w411
              tunnel: w408 -> [w414 w416]
              tunnel: w407 -> [w413 _]
              tunnel: w404 -> [w412 _]
              frame True {
                n147 = invoke class="VI" method="FP.Open"(reference=w413, error in=w414, "State"=w412) -> (error out=w415:errorcluster)  [unwired: 2 in, 4 out]
              }
              frame False {
              }
            }
          }
        }
        n148 = call <vilib>:"Add State(s) to Queue__JKI_lib_State_Machine.vi"("State(s) in (\"\")"=w351) -> ("States Out"=w350:string)  [unwired: 14 in]
      }
      frame "UI: Update Column Names" {
        n149 = Unbundle By Name(w418) -> ("JKISM Names"=w417:string[])
        n150 = property on="Table" class="Tbl (strict)"("Column Headers[]"=w417) -> ()  [unwired: 2 in, 2 out]
      }
      frame "UI: Update Content" {
        n151 = Unbundle By Name(w425) -> ("RowHeaders"=w423:string[], "Content"=w424:string[][])
        n152 = local write "Row Header Strings[]"(w423) -> ()
        n153 = local write "Content"(w424) -> ()
      }
      frame "UI: Autrosize Multilistbox Columns" {
        n154 = Unbundle By Name(w433) -> ("Content"=w432:string[][])  [unwired: 1 out]
        n155 = control-ref of="Table"() -> (w431:refnum<vi>)
        n156 = call "Auto Resize All MultiListbox Columns (Uniform Text).vi"("Array"=w432, "Control in"=w431) -> ("error out"=w430:errorcluster)  [unwired: 9 in]
      }
      frame "--------- Event ---------" {
      }
      frame "Register User Event" {
        n157 = call "CSM - Global Log Event.vi"() -> ("Error out"=w445:errorcluster, "CSM Global Log Event"=w442:refnum<user-event>)  [unwired: 10 in]
        n158 = register-events(error in=w445, w442) -> (reference out=w444:refnum<event-registration>)  [unwired: 1 in, 1 out]
        n159 = Bundle By Name(cluster=w447, "CSM Global Log Event"=w442) -> (w443:T6)
      }
      frame "UnRegister User Event" {
        n160 = Unregister For Events(event registration refnum=w454) -> (error out=w453:errorcluster)  [unwired: 1 in]
        n161 = Unbundle By Name(w452) -> ("CSM Global Log Event"=w451:refnum<user-event>)
        n162 = call "CSM - Destroy Global Log Event.vi"("Error in"=w453, "CSM Global Log Event"=w451) -> ("Error out"=w450:errorcluster)  [unwired: 9 in]
        n163 = call <vilib>:"Clear Errors.vi"("error in (no error)"=w450) -> ()  [unwired: 5 in, 2 out]
      }
      frame "---------- Macro ----------" {
        # "Do not put any code in this frame.\n(It is a separator no-op. You can make a copy of this frame to create a new Macro frame)"
        n164 = call <vilib>:"Add State(s) to Queue__JKI_lib_State_Machine.vi"("State(s) in (\"\")"=w463) -> ("States Out"=w462:string)  [unwired: 14 in]
      }
      frame "Macro: Initialize" {
        # "Initialization Macro\n(This is called once, when the VI starts)"
        n165 = call <vilib>:"Add State(s) to Queue__JKI_lib_State_Machine.vi"("State(s) in Front (\"\")"="Data: Initialize\nInitialize Core Data\nData: Load from INI\nUI: Initialize\nRegister User Event\n//UI: Front Panel State >> Open\nUI: Update Column Names\nUI: Update Content\nUI: Autrosize Multilistbox Columns", "State(s) in (\"\")"=w470) -> ("States Out"=w469:string)  [unwired: 13 in]
      }
      frame "Macro: UI Refresh" {
        # "Do not put any code in this frame.\n(It is a separator no-op. You can make a copy of this frame to create a new Macro frame)"
        n166 = call <vilib>:"Add State(s) to Queue__JKI_lib_State_Machine.vi"("State(s) at Back (\"\")"="UI: Update Column Names\nUI: Update Content" ("State(s) in Front (\"\")")) -> ("States Out"=w475:string)  [unwired: 14 in]
        n167 = call <vilib>:"Add State(s) to Queue__JKI_lib_State_Machine.vi"("State(s) in Front (\"\")"=w475, "State(s) in (\"\")"=w478) -> ("States Out"=w477:string)  [unwired: 13 in]
      }
      frame "Macro: Exit" {
        # "Exit Macro\n(This is called once, when the VI exits)"
        n168 = Unbundle By Name(w488) -> ("Core.Close Panel on Exit?"=w487:bool)
        n169 = Select(t="UI: Front Panel State >> Close", s=w487, f="") -> (s? t:f=w483:string)
        n170 = call <vilib>:"Add State(s) to Queue__JKI_lib_State_Machine.vi"("State(s) in Front (\"\")"="UnRegister User Event" ("State(s) in Front (\"\")"), "State(s) in (\"\")"=w483, "State(s) at Back (\"\")"="Data: Save to INI\nData: Cleanup\nExit") -> ("States Out"=w486:string)  [unwired: 12 in]
        n171 = call <vilib>:"Add State(s) to Queue__JKI_lib_State_Machine.vi"("State(s) in Front (\"\")"=w486, "State(s) in (\"\")"=w491) -> ("States Out"=w490:string)  [unwired: 13 in]
      }
      frame "----- Action ------" {
      }
      frame "Action: Clear Non-exist JKISM" {
        n172 = Get Variant Attribute(Variant=w518) -> (duplicate Variant=w517:variant, names=w515:string[], values=w514:variant[])  [unwired: 3 in, 1 out]
        n173 = Variant To Data(type=T4[] [], Variant=w514) -> (data=w513:T4[])  [unwired: 1 in, 1 out]
        n174 = Unbundle By Name(w511) -> ("Content"=w508:string[][], "JKISM Names"=w507:string[], "RowHeaders"=w501:string[])
        n175 = for {
          shift-right: [w546] -> w516
          shift-left: w517 -> [w547]
          tunnel: w515 -> [w545] mode=indexing
          tunnel: w513 -> [w544] mode=indexing
          tunnel: [w534] -> w510 mode=indexing if=w532
          n176 = Unbundle By Name(w544) -> ("Current State"=w542:string, "Name(\"\" to use uuid)"=w541:string)
          n177 = Search 1D Array(1D array=string[] ["<Remaining States>", "Exit"], element=w542) -> (index of element=w538:i32)  [unwired: 1 in]
          n178 = Match Pattern(string=w541, regular expression="^-") -> (offset past match=w539:i32)  [unwired: 1 in, 3 out]
          n179 = Greater Or Equal To 0?(x=w538) -> (x >= 0?=w536:bool)
          n180 = Greater Or Equal To 0?(x=w539) -> (x >= 0?=w537:bool)
          n181 = Or(x=w537, y=w536) -> (x .or. y?=w535:bool)
          n182 = case shown="True" w535 {
            tunnel: w547 -> [w548 w551]
            tunnel: [w548 w550] -> w546
            tunnel: w545 -> [_ w549]
            tunnel: w541 -> [_ _]
            tunnel: w542 -> [_ _]
            tunnel: [_ w549] -> w534
            frame False {
            }
            frame True {
              n183 = Delete Variant Attribute(6:w549, 7:w551) -> (3:w550:variant)  [unwired: 1 in, 2 out]
            }
          }
          n184 = Empty String/Path?(string/path=w534) -> (empty?=w533:bool)
          n185 = Not(x=w533) -> (.not. x?=w532:bool)
        }
        n186 = for {
          tunnel: w507 -> [w530] mode=indexing
          tunnel: w510 -> [w531]
          tunnel: [w529] -> w509 mode=indexing if=w527
          i -> [w529]
          n187 = Search 1D Array(1D array=w531, element=w530) -> (index of element=w528:i32)  [unwired: 1 in]
          n188 = Greater Or Equal To 0?(x=w528) -> (x >= 0?=w527:bool)
        }
        n189 = Reverse 1D Array(array=w509) -> (reversed array=w506:i32[])
        n190 = for {
          tunnel: w506 -> [w524] mode=indexing
          shift-right: [w523] -> w498
          shift-left: w508 -> [w526]
          shift-right: [w522] -> w504
          shift-left: w507 -> [w525]
          n191 = Delete From Array(array=w526, index (col)=w524) -> (array with subset deleted=w523:string[][])  [unwired: 2 in, 1 out]
          n192 = Delete From Array(array=w525, index=w524) -> (array with subset deleted=w522:string[])  [unwired: 1 in, 1 out]
        }
        n193 = Empty Array?(array=w498) -> (empty?=w499:bool)
        n194 = Select(t=string[] [] ("RowHeaders"), s=w499, f=w501) -> (s? t:f=w503:string[])
        n195 = Select(t=string[][] [] ("RowHeaders"), s=w499, f=w498) -> (s? t:f=w497:string[][])
        n196 = Bundle By Name(cluster=w511, "Content"=w497, "JKISM Names"=w504, "RowHeaders"=w503) -> (w505:T6)
      }
    }
  }
